vi "mult,div.vi"() -> ()   [LabVIEW 2020]
panel:
  in  "casos":T1(ring)=4
  in  "Numeric 3":dbl
  in  "Numeric 2":dbl
  out "Numeric":dbl
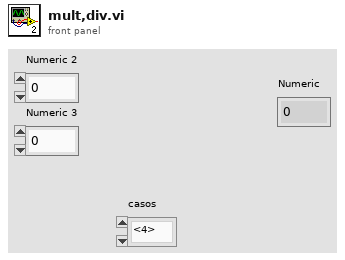
[diagram p1: front panel]
types:
  T1 = enum16{"divicion", "multiplicacion", "resta", "suma"}
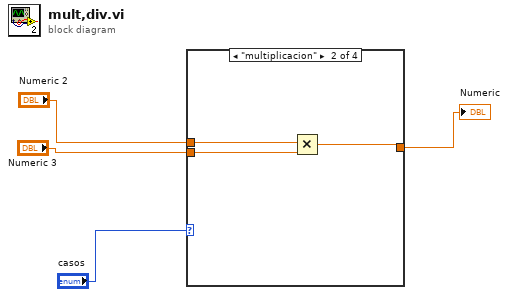
[diagram p0: block diagram]
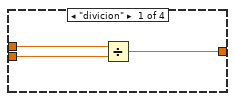
[diagram p2: hidden frame]
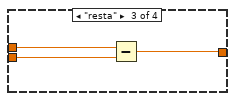
[diagram p3: hidden frame]
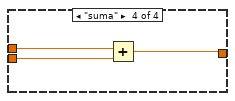
[diagram p4: hidden frame]
diagram:
  n1 = case shown="\"multiplicacion\"" "casos" {
    tunnel: "Numeric 2" -> [w7 w10 w13 w16]
    tunnel: "Numeric 3" -> [w6 w9 w12 w15]
    tunnel: [w5 w8 w11 w14] -> w1
    frame "divicion" {
      n2 = Divide(x=w7, y=w6) -> (x/y=w5:dbl)
    }
    frame "multiplicacion" {
      n3 = Multiply(x=w10, y=w9) -> (x*y=w8:dbl)
    }
    frame "resta" {
      n4 = Subtract(x=w13, y=w12) -> (x-y=w11:dbl)
    }
    frame "suma" {
      n5 = Add(x=w16, y=w15) -> (x+y=w14:dbl)
    }
  }
  "Numeric" <- w1
